vi "HW_Set_SYNC_Status.vi"(8 "error in (no error)":errorcluster, 9 "SYNC 2":bool, 10 "SYNC 1":bool, 11 "VISA Resource name IN":refnum<visa-resource-name>) -> (0 "error out":errorcluster, 3 "VISA resource name out":refnum<visa-resource-name>)   [LabVIEW 2018]
uses:
  <vilib>/Instr/_visa.llb/VISA Flush IO Buffer Mask.ctl
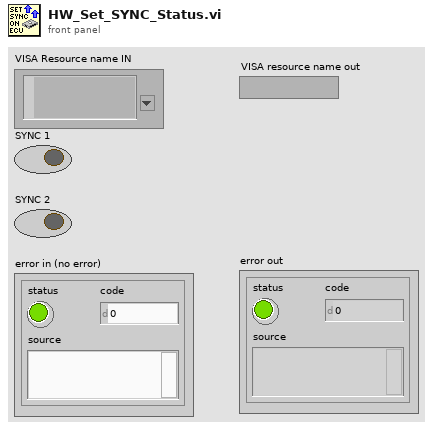
[diagram p1: front panel]
types:
  T1 = typedef "VISA Flush IO Buffer Mask.ctl" = u16
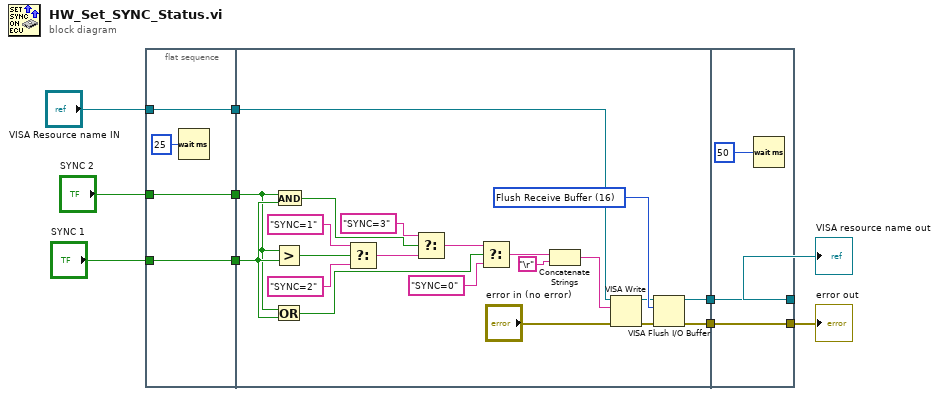
[diagram p0: block diagram]
diagram:
  n1 = flat-sequence {
    tunnel: "VISA Resource name IN" -> [w12]
    tunnel: "SYNC 2" -> [w13]
    tunnel: "SYNC 1" -> [w14]
    tunnel: [w14] -> w5
    tunnel: [w13] -> w4
    tunnel: [w12] -> w3
    tunnel: w5 -> [w20]
    tunnel: w4 -> [w19]
    tunnel: w3 -> [w18]
    tunnel: [w16] -> w2
    tunnel: [w15] -> w1
    tunnel: [w37] -> w6
    tunnel: [w38] -> w7
    tunnel: w2 -> [w38]
    tunnel: w1 -> [w37]
    frame #0 {
      n2 = Wait (ms)(milliseconds to wait=u32 25) -> ()  [unwired: 1 out]
    }
    frame #1 {
      w25 = T1 16 items=["Flush Receive Buffer"=16, "Write Transmit Buffer to Device"=32, "Flush Receive Buffer (No I/O)"=64, "Flush Transmit Buffer"=128] ("Mask")
      n3 = Greater?(x=w19, y=w20) -> (0:w29:bool)
      n4 = Or(x=w19, y=w20) -> (x .or. y?=w35:bool)
      n5 = And(x=w19, y=w20) -> (x .and. y?=w26:bool)
      n6 = Select(t="SYNC=1" ("string"), s=w29, f="SYNC=2" ("string")) -> (s? t:f=w31:string)
      n7 = Select(t="SYNC=3" ("string"), s=w26, f=w31) -> (s? t:f=w33:string)
      n8 = Select(t=w33, s=w35, f="SYNC=0") -> (s? t:f=w32:string)
      n9 = Concatenate Strings(w32, "\r") -> (w21:string)
      n10 = VISA Write(VISA resource name=w18, write buffer=w21, error in (no error)="error in (no error)") -> (VISA resource name out=w24:refnum<visa-resource-name>, error out=w23:errorcluster)  [unwired: 1 out]
      n11 = VISA Flush I/O Buffer(VISA resource name=w24, mask (16)=w25, error in (no error)=w23) -> (VISA resource name out=w16:refnum<visa-resource-name>, error out=w15:errorcluster)
    }
    frame #2 {
      n12 = Wait (ms)(milliseconds to wait=u32 50) -> ()  [unwired: 1 out]
    }
  }
  "VISA resource name out" <- w7
  "error out" <- w6
